vi "CMD_GOTOIF.vi"(8 "error in (no error)":errorcluster, 10 "Arguments":string[](array[string]), 11 "gScript Interpreter in":refnum<class "gScript Interpreter.lvclass">) -> (0 "error out":errorcluster, 3 "gScript Interpreter out":refnum<class "gScript Interpreter.lvclass">)   [LabVIEW 2017, in "gScript Interpreter.lvclass"]
uses:
  gScript Interpreter.lvclass
  gScript Interpreter.lvclass/gScript Interpreter.ctl
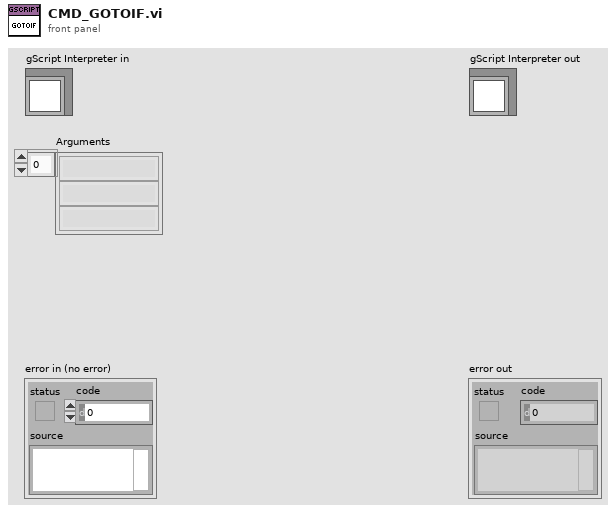
[diagram p1: front panel]
types:
  T1 = typedef "Memory Cell.ctl" = cluster{"type":T2, "x":dbl, "y":dbl, "z":dbl, "w":dbl}
  T2 = typedef "Memory Cell Type Enum.ctl" = enum16{"integer", "float", "vector", "rotation"}
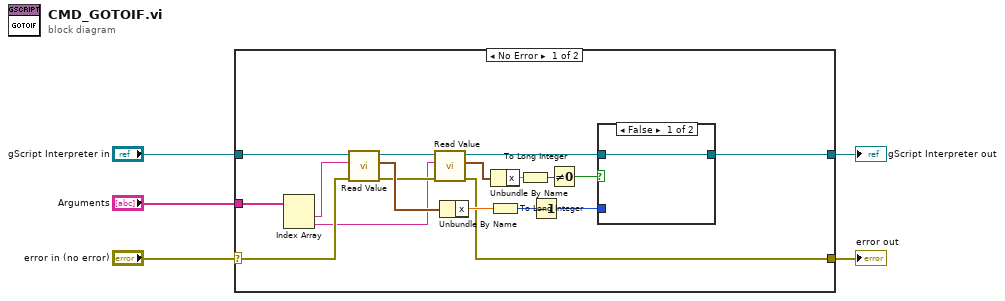
[diagram p0: block diagram]
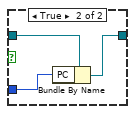
[diagram p2: hidden frame]
diagram:
  n1 = case shown="No Error" "error in (no error)" {
    selector: "error in (no error)" -> [w21 w29]
    tunnel: [w8 w29] -> w4
    tunnel: [w6 w28] -> w2
    tunnel: "gScript Interpreter in" -> [w22 w28]
    tunnel: "Arguments" -> [w23 _]
    frame No Error {
      n2 = Index Array(array=w23) -> (element #1=w20:string, element #2=w13:string)  [unwired: 2 in]
      n3 = call-dynamic "Read Value.vi"("error in (no error)"=w21, "String in"=w20, "gScript Interpreter in"=w22) -> ("error out"=w14:errorcluster, "Memory Cell"=w19:T1, "gScript Interpreter out"=w15:refnum<class "gScript Interpreter.lvclass">)  [unwired: 6 in]
      n4 = call-dynamic "Read Value.vi"("error in (no error)"=w14, "String in"=w13, "gScript Interpreter in"=w15) -> ("error out"=w8:errorcluster, "Memory Cell"=w12:T1, "gScript Interpreter out"=w7:refnum<class "gScript Interpreter.lvclass">)  [unwired: 6 in]
      n5 = Unbundle By Name(w19) -> ("x"=w18:dbl)
      n6 = To Long Integer(number=w18) -> (32bit integer=w17:i32)
      n7 = Unbundle By Name(w12) -> ("x"=w11:dbl)
      n8 = To Long Integer(number=w11) -> (32bit integer=w10:i32)
      n9 = Decrement(x=w17) -> (x-1=w16:i32)
      n10 = Not Equal To 0?(x=w10) -> (x != 0?=w9:bool)
      n11 = case shown="False" w9 {
        tunnel: w16 -> [_ w27]
        tunnel: w7 -> [w24 w26]
        tunnel: [w24 w25] -> w6
        frame False {
        }
        frame True {
          n12 = Bundle By Name(cluster=w26, "PC"=w27) -> (w25:refnum<class "gScript Interpreter.lvclass">)
        }
      }
    }
    frame Error {
    }
  }
  "error out" <- w4
  "gScript Interpreter out" <- w2
